vi "Get top-level path.vi"() -> (1 "Top-level LabVIEW path":path)   [LabVIEW 2012]
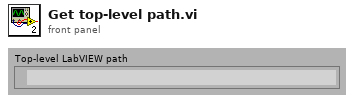
[diagram p1: front panel]
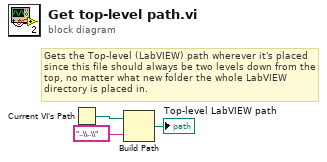
[diagram p0: block diagram]
diagram:
  # "Gets the Top-level (LabVIEW) path wherever it's placed\nsince this file should always be two levels down from the \ntop, no matter what new folder the whole LabVIEW\ndirectory is placed in."
  n1 = Current VI's Path() -> (path=w2:path)
  n2 = Build Path(base path=w2, name or relative path="..\\..\\") -> (appended path=→"Top-level LabVIEW path":path)
